vi "Post-Build Action.vi"(5 "Files Generated by Build":path[](array[path]), 6 "Top Level/Always Included VIs":path[](array[path]), 7 "Destination Path":path, 8 "error in (no error)":errorcluster, 9 "Target Name":string, 10 "Build Specification Name":string, 11 "Project Path":path) -> (0 "error out":errorcluster)   [LabVIEW 2014]
uses:
  <vilib>/Utility/config.llb/Write Key (Boolean).vi
  <vilib>/Utility/config.llb/NI_LVConfig.lvlib
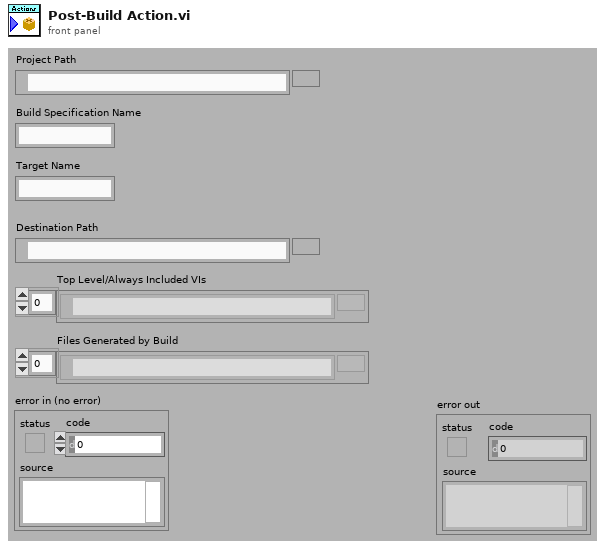
[diagram p1: front panel]
types:
  T1 = typedef "NI_LVConfig.lvlib/Config Data RefNum.ctl" = refnum<k1>
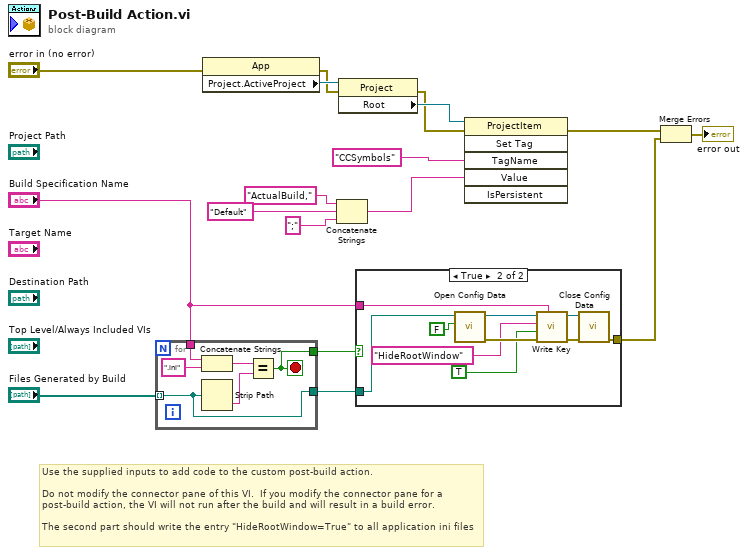
[diagram p0: block diagram]
diagram:
  # "Use the supplied inputs to add code to the custom post-build action.\n\nDo not modify the connector pane of this VI.  If you modify the connector pane for a post-build action, the VI will not run after the build and will result in a build error.\n\nThe second part should write the entry \"HideRootWindow=True\" to all application ini files"
  n1 = for {
    tunnel: "Files Generated by Build" -> [w19] mode=indexing
    tunnel: "Build Specification Name" -> [w23]
    tunnel: [w19] -> w8
    tunnel: [w18] -> w7
    stop <- w18 stop-if-true
    n2 = Concatenate Strings(w23, ".ini" ("string")) -> (w20:string)
    n3 = Strip Path(path=w19) -> (name=w21:string)  [unwired: 1 out]
    n4 = Equal?(x=w20, y=w21) -> (x = y?=w18:bool)
  }
  n5 = property class="App"(error in="error in (no error)") -> (error out=w5:errorcluster, "Project.ActiveProject"=w17:refnum<vi>)  [unwired: 1 in, 1 out]
  n6 = Concatenate Strings("ActualBuild," ("Tag Name"), "Default" ("Tag Name"), ";" ("string")) -> (w11:string)
  n7 = property class="Project"(reference=w17, error in=w5) -> (error out=w4:errorcluster, "Root"=w16:refnum<vi>)  [unwired: 1 out]
  n8 = case shown="True" w7 {
    tunnel: "Build Specification Name" -> [_ w26]
    tunnel: w8 -> [_ w25]
    tunnel: [_ w24] -> w1
    frame False {
    }
    frame True {
      n9 = call <vilib>:"Open Config Data.vi"("create file if necessary (T)"=FALSE, "configuration file path"=w25) -> ("error out"=w33:errorcluster, "refnum"=w30:T1)  [unwired: 7 in, 1 out]
      n10 = call-poly <vilib>:"Write Key.vi"("section"=w26, "error in (no error)"=w33, "value"=TRUE, "key"="HideRootWindow", "refnum"=w30) -> ("error out"=w32:errorcluster, "refnum out"=w31:T1)  [unwired: 4 in, 1 out]
      n11 = call <vilib>:"Close Config Data.vi"("error in (no error)"=w32, "refnum"=w31) -> ("error out"=w24:errorcluster)  [unwired: 8 in, 1 out]
    }
  }
  n12 = invoke class="ProjectItem" method="Set Tag"(reference=w16, error in=w4, "TagName"="CCSymbols" ("Tag Name"), "Value"=w11) -> (error out=w3:errorcluster)  [unwired: 2 in, 5 out]
  n13 = Merge Errors(w3, w1) -> (→"error out":errorcluster)
